vi "Read Configuration Parameters.vi"(8 "error in (no error)":errorcluster, 10 "refnum":T1, 11 "VacuumLine Configuration in":refnum<class "VacuumLine Configuration.lvclass">) -> (0 "error out":errorcluster, 2 "refnum out":T1, 3 "VacuumLine Configuration out":refnum<class "VacuumLine Configuration.lvclass">)   [LabVIEW 2016, in "Hardware.lvlib" / "VacuumLine.lvlib" / "VacuumLine Configuration.lvclass"]
uses:
  <userlib>/Common Components/Hardware/Abstract System/VacuumLine/VacuumLine Config/VacuumLine Configuration.lvclass
  <vilib>/Utility/config.llb/Config Data RefNum.ctl
  <userlib>/Common Components/Hardware/Abstract System/VacuumLine/VacuumLine Config/VacuumLine Configuration.lvclass/VacuumLine Configuration.ctl
  <userlib>/Common Components/Hardware/Abstract System/VacuumLine/VacuumLine/VacuumLine.lvclass/VacuumLine.ctl
  <userlib>/Common Components/Hardware/Abstract System/VacuumLine/VacuumLine/Read VacuumLine Params.vi
  <userlib>/Common Components/Hardware/Abstract System/VacuumLine/VacuumLine/Write VacuumLine Params.vi
  <userlib>/Common Components/Hardware/Abstract System/VacuumLine/VacuumLine/Read Array of Move Button Configurations.vi
  <userlib>/Common Components/Hardware/Abstract System/VacuumLine/VacuumLine/Write Array of Move Button Configurations.vi
  <userlib>/Configuration Dialog Actor/Configuration.lvclass
  <userlib>/Common Components/Hardware/Motor/Motor Config/Motor Configuration.lvclass
  <vilib>/Utility/config.llb/NI_LVConfig.lvlib
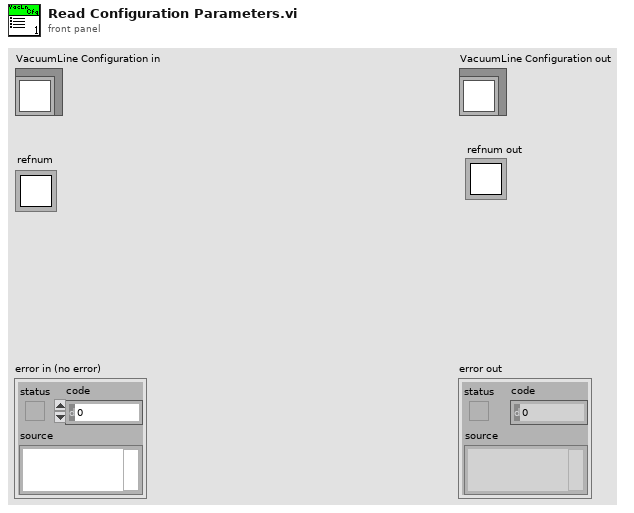
[diagram p1: front panel]
types:
  T1 = typedef "NI_LVConfig.lvlib/Config Data RefNum.ctl" = refnum<k1>
  T2 = typedef "Hardware.lvlib/VacuumLine.lvlib/VacuumLine.lvclass/VacuumLine Params.ctl" = cluster{"Motion Limits":cluster{"min":dbl, "max":dbl}, "No. of Conflict Zones":u8, "Conflict Zones (mm)":cluster{"with":string, "from":dbl, "to":dbl, "buffer":dbl}[], "Valve Complexes":T3[], "max( |Motor Pos - LRF Distance| )":dbl}
  T3 = typedef "Hardware.lvlib/VacuumLine.lvlib/VacuumLine.lvclass/Valve Complex.ctl" = cluster{"LogicIO Module":string, "Valve Open":T4, "Optical Switch -":T4, "Optical Switch +":T4, "Valve Closed Status Alert":cluster{"Pin#":u8, "Option":enum16{"Not Used", "Normally Closed"}}}
  T4 = typedef "Hardware.lvlib/VacuumLine.lvlib/VacuumLine.lvclass/Logic Cluster.ctl" = cluster{"Pin#":u8, "Location":dbl, "Tolerance":dbl}
  T5 = typedef "Hardware.lvlib/VacuumLine.lvlib/VacuumLine.lvclass/Button Config Cluster.ctl" = cluster{"Enabled?":bool, "Text on button":string, "Target pos":dbl}
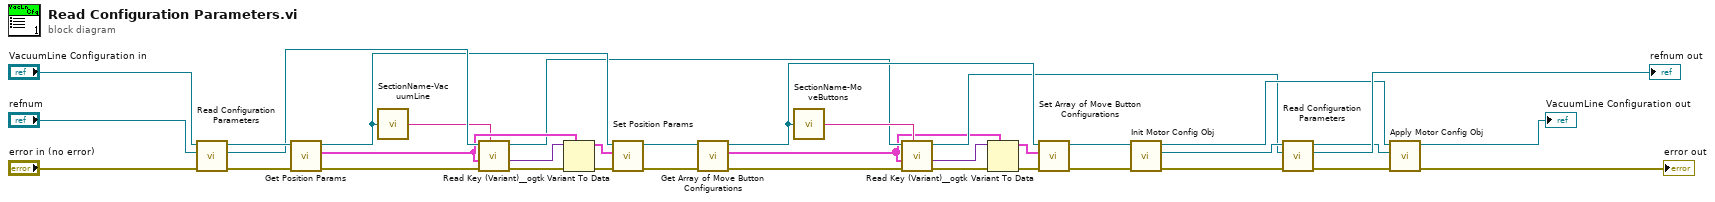
[diagram p0: block diagram]
diagram:
  n1 = call-parent "Read Configuration Parameters.vi"("error in (no error)"="error in (no error)", "refnum"="refnum", "Configuration in"="VacuumLine Configuration in") -> ("error out"=w32:errorcluster, "refnum out"=w26:T1, "Configuration out"=w30:refnum<class "VacuumLine Configuration.lvclass">)  [unwired: 6 in]
  n2 = call <userlib>:"Get Position Params.vi"("error in (no error)"=w32, "VacuumLine Configuration in"=w30) -> ("error out"=w31:errorcluster, "Position Params"=w24:T2, "VacuumLine Configuration out"=w20:refnum<class "VacuumLine Configuration.lvclass">)  [unwired: 7 in]
  n3 = call <userlib>:"SectionName-VacuumLine.vi"("VacuumLine Configuration in"=w20) -> ("SectionName"=w21:string)
  n4 = call <userlib>:"Read Key (Variant)__ogtk.vi"("section"=w21, "error in (no error)"=w31, "type"=w24, "refnum"=w26) -> ("error out"=w27:errorcluster, "key-value"=w23:variant, "refnum out"=w5:T1)  [unwired: 4 in, 1 out]
  n5 = Variant To Data(error in=w27, type=w24, Variant=w23) -> (data=w22:T2, error out=w25:errorcluster)
  n6 = call <userlib>:"Set Position Params.vi"("error in (no error)"=w25, "Position Params"=w22, "VacuumLine Configuration in"=w20) -> ("error out"=w28:errorcluster, "VacuumLine Configuration out"=w12:refnum<class "VacuumLine Configuration.lvclass">)  [unwired: 7 in]
  n7 = call <userlib>:"Get Array of Move Button Configurations.vi"("error in (no error)"=w28, "VacuumLine Configuration in"=w12) -> ("error out"=w13:errorcluster, "Array of Move Button Configurations"=w3:T5[], "VacuumLine Configuration out"=w9:refnum<class "VacuumLine Configuration.lvclass">)  [unwired: 7 in]
  n8 = call <userlib>:"SectionName-MoveButtons.vi"("VacuumLine Configuration in"=w9) -> ("SectionName"=w6:string)
  n9 = call <userlib>:"Read Key (Variant)__ogtk.vi"("section"=w6, "error in (no error)"=w13, "type"=w3, "refnum"=w5) -> ("error out"=w8:errorcluster, "key-value"=w2:variant, "refnum out"=w4:T1)  [unwired: 4 in, 1 out]
  n10 = Variant To Data(error in=w8, type=w3, Variant=w2) -> (data=w1:T5[], error out=w7:errorcluster)
  n11 = call <userlib>:"Set Array of Move Button Configurations.vi"("error in (no error)"=w7, "Array of Move Button Configurations"=w1, "VacuumLine Configuration in"=w9) -> ("error out"=w11:errorcluster, "VacuumLine Configuration out"=w10:refnum<class "VacuumLine Configuration.lvclass">)  [unwired: 7 in]
  n12 = call <userlib>:"Init Motor Config Obj.vi"("error in (no error)"=w11, "VacuumLine Configuration in"=w10) -> ("error out"=w19:errorcluster, "Motor Config Obj"=w15:refnum<class "Motor Configuration.lvclass">, "VacuumLine Configuration out"=w18:refnum<class "VacuumLine Configuration.lvclass">)  [unwired: 7 in]
  n13 = call-dynamic "Read Configuration Parameters.vi"("error in (no error)"=w19, "refnum"=w4, "Example Configuration Dialog in"=w15) -> ("error out"=w29:errorcluster, "refnum out"=→"refnum out":T1, "Example Configuration Dialog out"=w14:refnum<class "Motor Configuration.lvclass">)  [unwired: 6 in]
  n14 = call <userlib>:"Apply Motor Config Obj.vi"("error in (no error)"=w29, "Motor Config Obj"=w14, "VacuumLine Configuration in"=w18) -> ("error out"=→"error out":errorcluster, "VacuumLine Configuration out"=→"VacuumLine Configuration out":refnum<class "VacuumLine Configuration.lvclass">)  [unwired: 7 in]
